vi "FL_ZLEMA_Filter.vi"(1 "EMA filter coefficients":dbl[](array[numeric]), 2 "Initialize? (F)":bool, 3 "Input X":sgl) -> (0 "Filtered X":dbl)   [LabVIEW 2018, in "Tracker.lvlib"]
uses:
  Tracker.lvlib
  <vilib>/ptbypt/NI_PtbyPt.lvlib
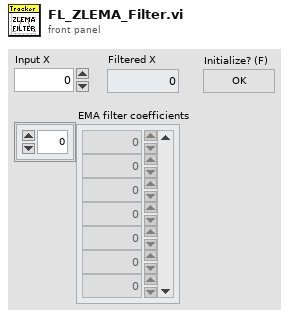
[diagram p1: front panel]
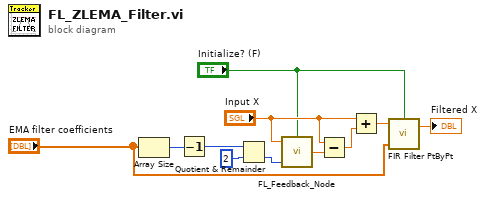
[diagram p0: block diagram]
diagram:
  n1 = Array Size(array="EMA filter coefficients") -> (size(s)=w6:i32)
  n2 = Decrement(x=w6) -> (x-1=w5:i32)
  n3 = Quotient & Remainder(x=w5, y=2) -> (floor(x/y)=w3:i32)  [unwired: 1 out]
  n4 = call "FL_Feedback_Node.vi"("Reset Node"="Initialize? (F)", "Delay"=w3, "Input X"="Input X") -> ("Delayed X"=w8:dbl)  [unwired: 1 in]
  n5 = Subtract(x="Input X", y=w8) -> (x-y=w9:dbl)
  n6 = Add(x="Input X", y=w9) -> (x+y=w11:dbl)
  n7 = call <vilib>:"FIR Filter PtByPt.vi"("initialize"="Initialize? (F)", "Forward Coefficients"="EMA filter coefficients", "x"=w11) -> ("Filtered x"=→"Filtered X":dbl)  [unwired: 1 in, 1 out]
